vi "verify client optionally.vi"(8 "error in":errorcluster, 11 "lvlibretls server listener in":refnum<class "lvlibretls server listener.lvclass">) -> (0 "error out":errorcluster, 3 "lvlibretls server listener out":refnum<class "lvlibretls server listener.lvclass">)   [LabVIEW 2016, in "lvlibretls server listener.lvclass"]
uses:
  lvlibretls server listener.lvclass
  C:/Users/IEUser/Desktop/tlssimple/libretls/context parent/lvlibretls configurable context.lvclass
  context parent/lvlibretls configurable context.lvclass/lvlibretls configurable context.ctl
  context parent/lvlibretls configurable context.lvclass
  lv tls dll.lvlib
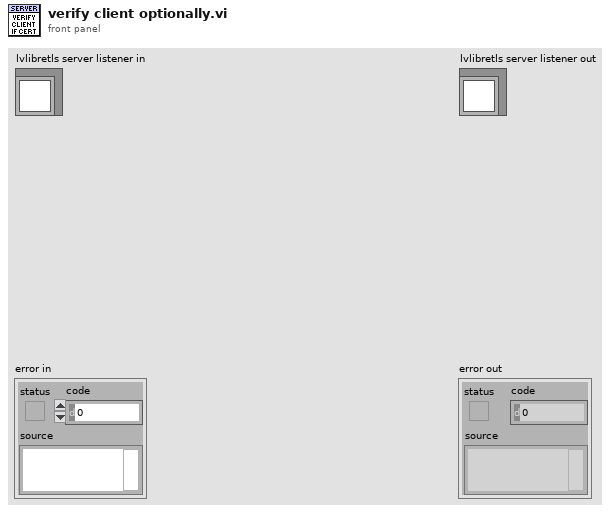
[diagram p1: front panel]
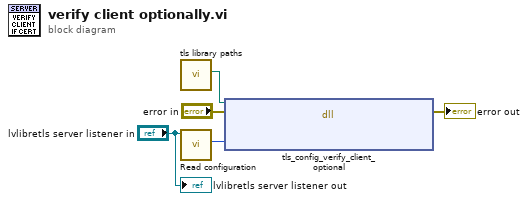
[diagram p0: block diagram]
diagram:
  n1 = call "tls library paths.vi"() -> ("libtls"=w4:path)  [unwired: 8 in, 3 out]
  n2 = call "Read configuration.vi"("lvlibretls configurable context in"="lvlibretls server listener in") -> ("configuration"=w2:u64)  [unwired: 10 in]
  n3 = dll-call lib="C:/Users/IEUser/Desktop/tlssimple/libtls-15.dll" fn="tls_config_verify_client_optional"(path in=w4, error in="error in", "config"=w2) -> (error out=→"error out":errorcluster)  [unwired: 3 in, 1 out]
  "lvlibretls server listener out" <- "lvlibretls server listener in"
